vi "filterSQL.vi"(5 "Experiment":u16(ring) items=["10TW", "test stand", "LaserUpstairs", "Staging"]) -> (0 "filtered":string[](array[string]), 2 "data":string[][](array[string]))   [LabVIEW 2013]
uses:
  Shared/MySQL/Preset Query Enum.ctl
  <userlib>/_OpenG.lib/array/array.llb/Filter 1D Array with Scalar (String)__ogtk.vi
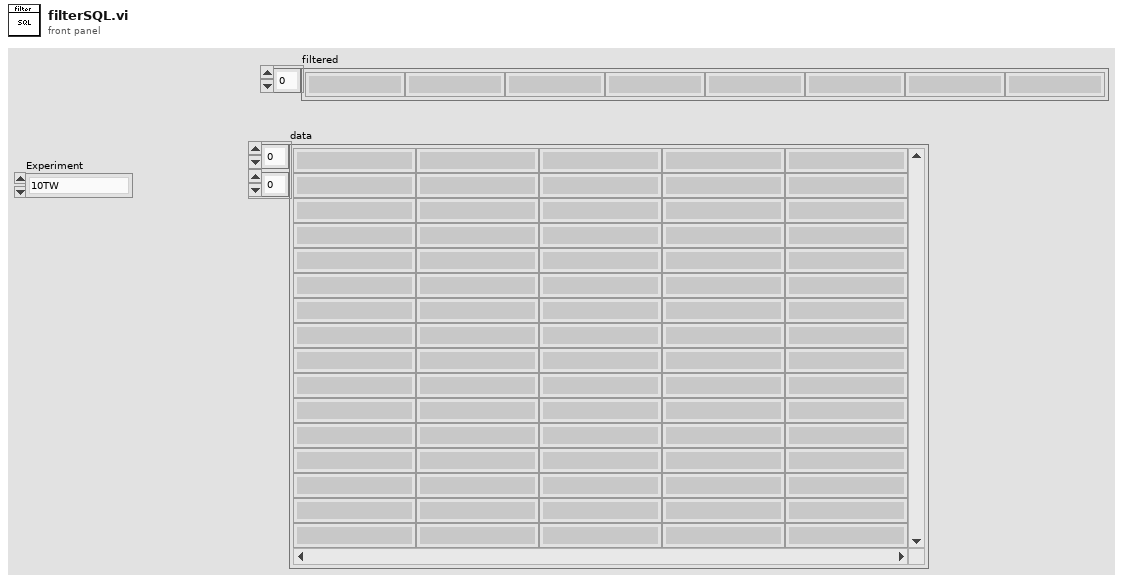
[diagram p1: front panel]
types:
  T1 = typedef "Preset Query Enum.ctl" = enum16{"Get Locations", "Get all IPs and MACs", "Get classes", "Get expt variables to set at scanstart for particular device", "Get expt devices and variables with start values", "Get expt devices and variables (with data to get)", "Get expt devices with data to get", "Get Expt devices and GUIs", "Get all devices basic properties", "Get Virtual Devices Core Info", "Get Expt names", "Get experiment basic properties", "Get experiment alarm variables", "Get MC Ports", "Get device network comm port", "Get devicetype lvclass path", "Get basic device properties", "Get Init Order", "Get all setable variables of a device", "Get device variable aliases", "Get force values of all settable variables", "Get all variables of a devicetype", "Get all variables of a device", "Get plotter details", "Get Saved Scans", "Get Scan Info", "GetGeneralGUIs", "Get expt for plotter", "Get plotter IDs from expt", "Get all devices", "Get all Virtual Devices", "Get all aliases", "Get variable and device info for Virtual Device", "GetItemLocatorIP", "Get IPs for GUIs", "Get DeviceType from Device", "GetLocalPortRange", "GetDevicePresetVariables", "Get Device Configuration", "GetAllPresetNames", "GetAllConfigurationNames", "GetPresetDeviceNames"}
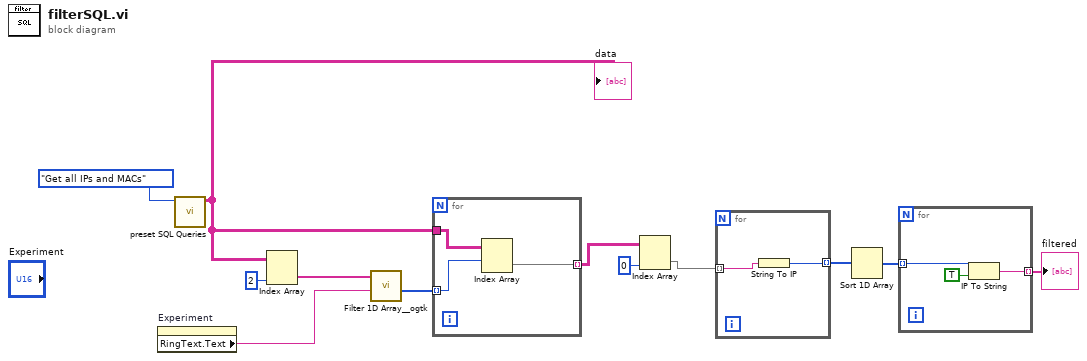
[diagram p0: block diagram]
diagram:
  n1 = property on="Experiment" class="Ring (strict)"() -> ("RingText.Text"=w8:string)  [unwired: 2 in, 2 out]
  n2 = call "preset SQL Queries.vi"("Preset Query"=Preset_Query_Enum."Get all IPs and MACs") -> ("data"=w7:string[][])  [unwired: 8 in, 2 out]
  "data" <- w7
  n3 = Index Array(array=w7, index (col)=2 ("disabled index (col)")) -> (element=w10:string[])  [unwired: 1 in]
  n4 = call-poly <userlib>:"Filter 1D Array__ogtk.vi"("items to filter"=w8, "array"=w10) -> ("filtered item indices"=w9:i32[])  [unwired: 4 in, 1 out]
  n5 = for {
    tunnel: w9 -> [w14] mode=indexing
    tunnel: w7 -> [w15]
    tunnel: [w13] -> w6 mode=indexing
    n6 = Index Array(array=w15, index (row)=w14) -> (element=w13:string[])  [unwired: 1 in]
  }
  n7 = Index Array(array=w6, index (col)=0 ("disabled index (col)")) -> (element=w3:string[])  [unwired: 1 in]
  n8 = for {
    tunnel: [w17] -> w5 mode=indexing
    tunnel: w3 -> [w16] mode=indexing
    n9 = String To IP(1:w16) -> (0:w17:u32)
  }
  n10 = Sort 1D Array(array=w5) -> (sorted array=w2:u32[])
  n11 = for {
    tunnel: w2 -> [w19] mode=indexing
    tunnel: [w18] -> w1 mode=indexing
    n12 = IP To String(1:TRUE ("dot notation? (F)"), 2:w19) -> (0:w18:string)
  }
  "filtered" <- w1
